vi "Write Result Channel Refs.vi"(8 "error in (no error)":errorcluster, 10 "Result Channel Refs":T1[](array[typedef]) format="%.0x", 11 "WaveformCalculation in":refnum<class "WaveformCalculation.lvclass">) -> (0 "error out":errorcluster, 3 "WaveformCalculation out":refnum<class "WaveformCalculation.lvclass">)   [LabVIEW 2015, in "WaveformCalculation.lvclass"]
uses:
  WaveformCalculation.lvclass
  <vilib>/NI Veristand/Custom Device API/Custom Device Item Ref.ctl
  WaveformCalculation.lvclass/WaveformCalculation.ctl
  <vilib>/NI VeriStand/Custom Device API/Custom Device API.lvlib
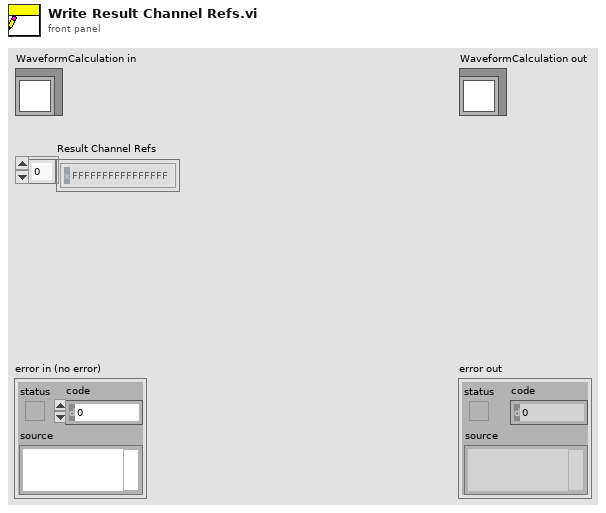
[diagram p1: front panel]
types:
  T1 = typedef "Custom Device API.lvlib/Custom Device Item Ref.ctl" = u64
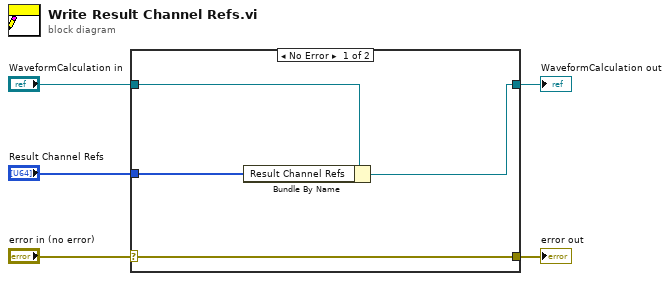
[diagram p0: block diagram]
diagram:
  n1 = case shown="No Error" "error in (no error)" {
    selector: "error in (no error)" -> [w9 w10]
    tunnel: [w9 w10] -> w4
    tunnel: [w7 w11] -> w2
    tunnel: "WaveformCalculation in" -> [w8 w11]
    tunnel: "Result Channel Refs" -> [w6 _]
    frame No Error {
      n2 = Bundle By Name(cluster=w8, "Result Channel Refs"=w6) -> (w7:refnum<class "WaveformCalculation.lvclass">)
    }
    frame Error {
    }
  }
  "error out" <- w4
  "WaveformCalculation out" <- w2
